vi "Heater Control.vi"(0 "Heater Level":enum16{"Off", "Medium", "Maximum"}(ring)) -> (3 "Heater Level (V)":dbl format="%#.3f", 4 "error out":errorcluster)   [LabVIEW 2024]
uses:
  <vilib>/Utility/error.llb/DialogType.ctl
  <vilib>/DAQmx/write.llb/DAQmx Write (Analog DBL 1Chan 1Samp).vi
  <vilib>/DAQmx/read.llb/DAQmx Read (Analog DBL 1Chan 1Samp).vi
  <vilib>/DAQmx/create/channels.llb/DAQmx Create Channel (AO-Voltage-Basic).vi
  <vilib>/DAQmx/create/channels.llb/DAQmx Create Channel (AI-Voltage-Basic).vi
  <vilib>/DAQmx/miscellaneous.llb/DAQmx Fill In Error Info.vi
panel:
  in  "error in (no error)":errorcluster
  in  "input terminal configuration":i32(ring)=10083 items=["Default"=-1, "RSE"=10083, "NRSE"=10078, "Differential"=10106, "Pseudodifferential"=12529]
  in  "physical input channels":tag="Dev1/ai1"
  in  "physical output channel":tag="Dev1/ao0"
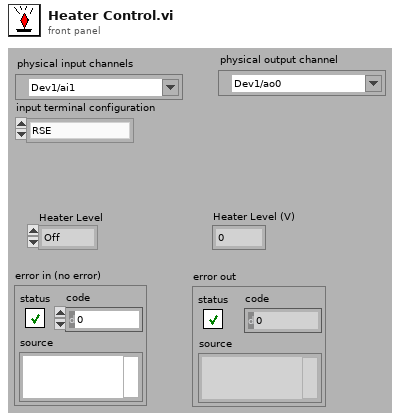
[diagram p1: front panel]
types:
  T1 = typedef "DialogType.ctl" = u16
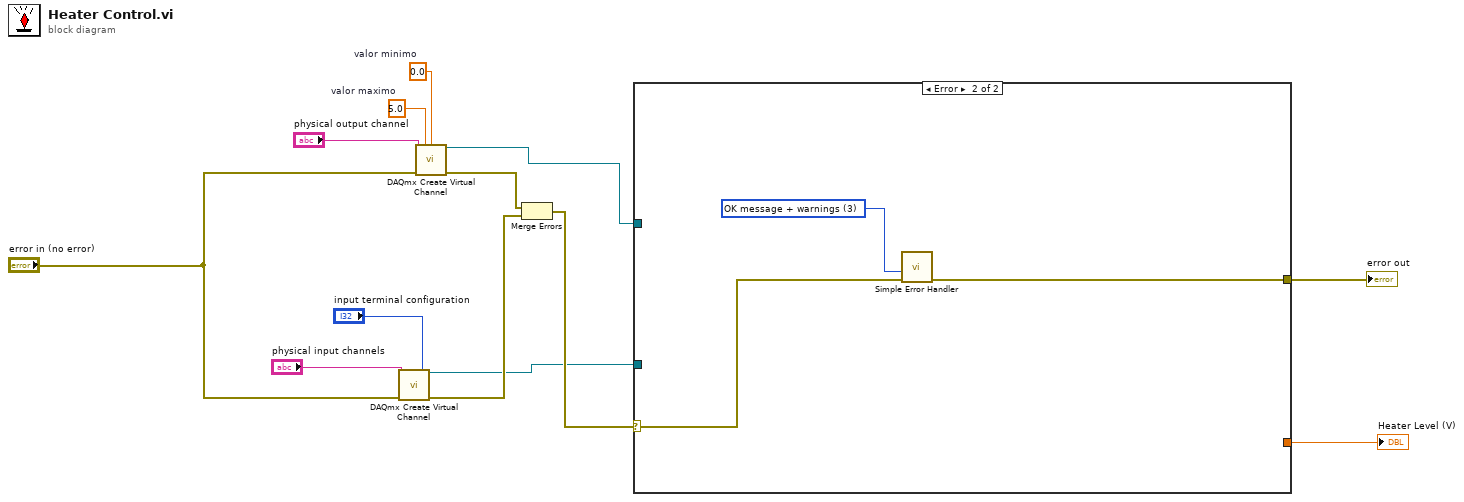
[diagram p0: block diagram]
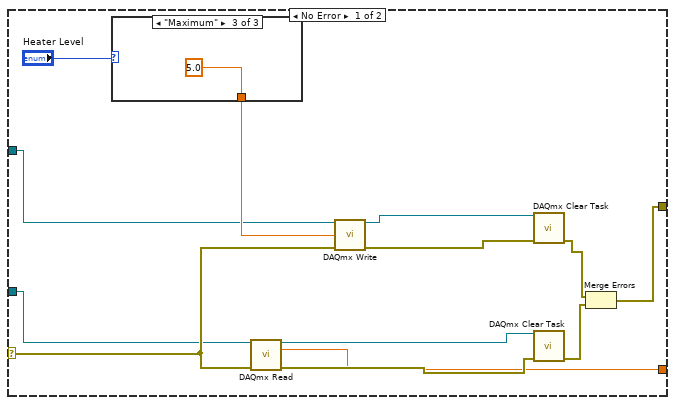
[diagram p2: hidden frame]
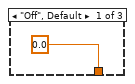
[diagram p3: hidden frame]
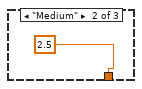
[diagram p4: hidden frame]
diagram:
  w11 = 0.0  # valor minimo
  w12 = 5.0  # valor maximo
  n1 = call-poly <vilib>:"DAQmx Create Virtual Channel.vi"("input terminal configuration"="input terminal configuration", "physical channels"="physical input channels", "error in"="error in (no error)") -> ("task out"=w3:refnum<k21>, "error out"=w9:errorcluster)  [unwired: 11 in]
  n2 = call-poly <vilib>:"DAQmx Create Virtual Channel.vi"("maximum value"=w12, "minimum value"=w11, "physical channels"="physical output channel", "error in"="error in (no error)") -> ("task out"=w2:refnum<k21>, "error out"=w10:errorcluster)  [unwired: 10 in]
  n3 = Merge Errors(w10, w9) -> (w4:errorcluster)
  n4 = case shown="Error" w4 {
    selector: w4 -> [w17 w31]
    tunnel: [w19 w32] -> w13
    tunnel: w3 -> [w16 _]
    tunnel: w2 -> [w15 _]
    tunnel: [w14 _] -> w1
    frame No Error {
      n5 = case shown="\"Maximum\"" "Heater Level" {
        tunnel: [0.0 2.5 5.0] -> w26
        frame "Off", Default {
        }
        frame "Medium" {
        }
        frame "Maximum" {
        }
      }
      n6 = call-poly <vilib>:"DAQmx Read.vi"("task/channels in"=w16, "error in"=w17) -> ("task out"=w23:refnum<k21>, "data"=w14:dbl, "error out"=w22:errorcluster)  [unwired: 11 in]
      n7 = call-poly <vilib>:"DAQmx Write.vi"("task/channels in"=w15, "data"=w26, "error in"=w17) -> ("task out"=w21:refnum<k21>, "error out"=w20:errorcluster)  [unwired: 10 in, 1 out]
      n8 = call <vilib>:"DAQmx Clear Task.vi"("task in"=w21, "error in"=w20) -> ("error out"=w24:errorcluster)  [unwired: 13 in]
      n9 = call <vilib>:"DAQmx Clear Task.vi"("task in"=w23, "error in"=w22) -> ("error out"=w25:errorcluster)  [unwired: 13 in]
      n10 = Merge Errors(w24, w25) -> (w19:errorcluster)
    }
    frame Error {
      w30 = T1 3 items=["no dialog", "OK message", "continue or stop message", "OK message + warnings", "continue/stop + warnings"] ("type of dialog (OK msg:1)")
      n11 = call <vilib>:"Simple Error Handler.vi"("type of dialog (OK msg:1)"=w30, "error in (no error)"=w31) -> ("error out"=w32:errorcluster)  [unwired: 3 in, 4 out]
    }
  }
  "error out" <- w13
  "Heater Level (V)" <- w1
